vi "Get ControlIndex.vi"(8 "error in (no error)":errorcluster, 11 "Terminal in":refnum<class "Terminal.lvclass">) -> (0 "error out":errorcluster, 2 "ControlIndex":i32, 3 "Terminal out":refnum<class "Terminal.lvclass">)   [LabVIEW 2021, in "smo.lvlib" / "Terminal.lvclass"]
uses:
  Terminal.lvclass
  Terminal.lvclass/Terminal.ctl
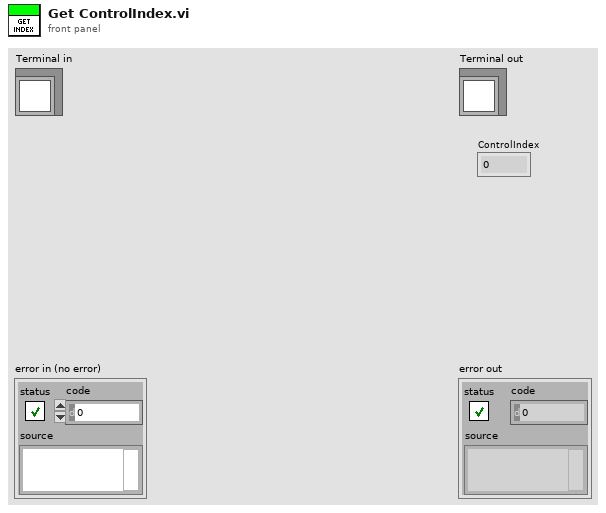
[diagram p1: front panel]
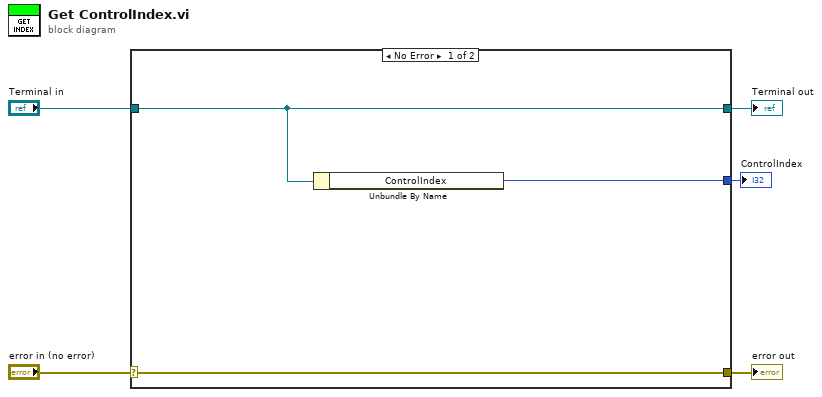
[diagram p0: block diagram]
diagram:
  n1 = case shown="No Error" "error in (no error)" {
    selector: "error in (no error)" -> [w8 w10]
    tunnel: [w8 w10] -> w4
    tunnel: [w7 w9] -> w2
    tunnel: "Terminal in" -> [w7 w9]
    tunnel: [w6 _] -> w1
    frame No Error {
      n2 = Unbundle By Name(w7) -> ("ControlIndex"=w6:i32)
    }
    frame Error {
    }
  }
  "error out" <- w4
  "Terminal out" <- w2
  "ControlIndex" <- w1
